vi "ViewData.vi"(7 "LabVIEW Web Service Request":refnum<class "Web Request.lvclass">) -> ()   [LabVIEW 2019]
uses:
  private/SendOutputDataState.ctl
  MobileAnalyzer/mainVIs/UIVIs/UIOutput.ctl
  MobileAnalyzer/mainVIs/analyzeAccelerationDataVIs/AccelerationDataFrames.ctl
  MobileAnalyzer/mainVIs/communicateWebServicesVIs/WebServicesData.ctl
  <vilib>/dex/Stream Element Allocation Mode.ctl
  <vilib>/wsapi/Web Request.lvclass
panel:
  # "Use the Web Service Request input terminal to call the VIs on the Web Services palette. Do not remove it from the connector pane unless you don't need access to the palette."
  # "Each additional control wired to the connector pane will be available as an input in the URL. To include an indicator in terminal-mode output (the default setting), it must also be wired to the connector pane."
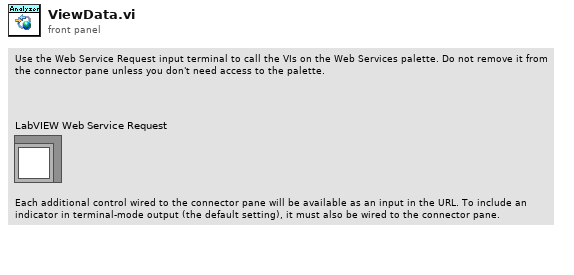
[diagram p1: front panel]
types:
  T1 = typedef "SendOutputDataState.ctl" = enum16{"Create analyzer endpoint", "Send output data", "End", "Init"}
  T2 = typedef "WebServicesData.ctl" = cluster{"AccelerationDataFrames":T3, "UIOutput":T4}
  T3 = typedef "AccelerationDataFrames.ctl" = cluster{"AccelerationData":waveform(dbl)[], "Amplitudes":cluster{"f0":dbl, "df":dbl, "real part":dbl[]}[], "Phases":cluster{"f0":dbl, "df":dbl, "imaginary part":dbl[]}[]}
  T4 = typedef "UIOutput.ctl" = cluster{"Aquiring data":bool, "AnalyzerError":errorcluster, "FIFO overflow":bool, "Analyzing data":bool}
  T5 = typedef "Stream Element Allocation Mode.ctl" = u32
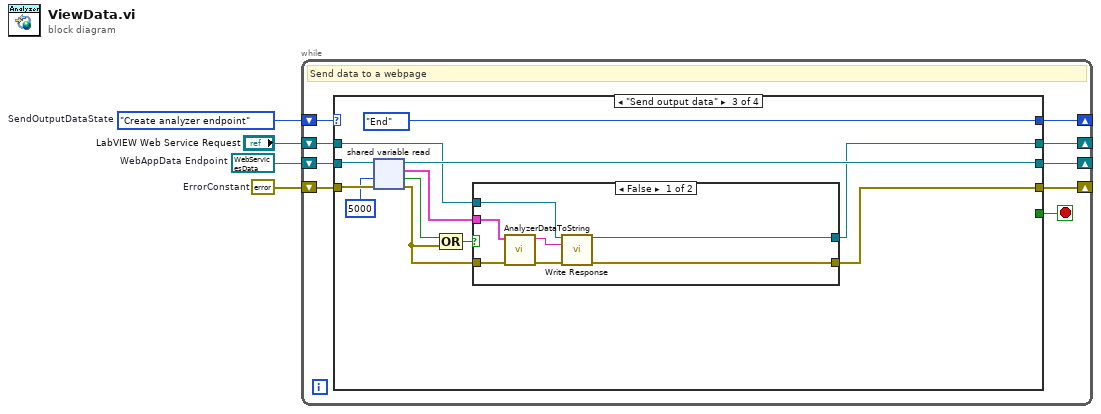
[diagram p0: block diagram]
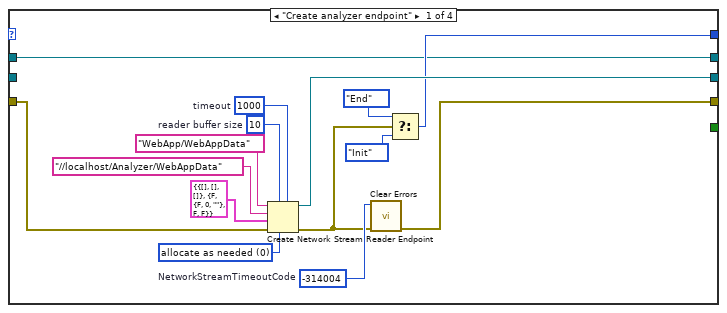
[diagram p2: hidden frame]
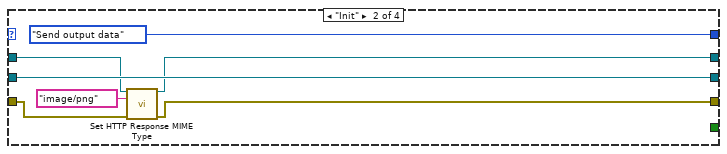
[diagram p3: hidden frame]
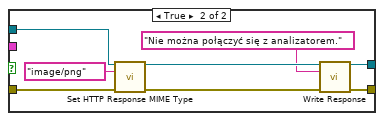
[diagram p4: hidden frame]
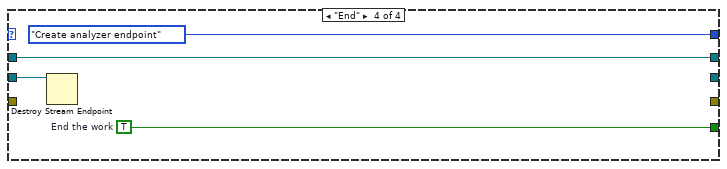
[diagram p5: hidden frame]
diagram:
  w2 = errorcluster {"status"=FALSE, "code"=0, "source"=""}  # ErrorConstant
  w3 = refnum<k21> refnum  # WebAppData Endpoint
  w4 = SendOutputDataState."Create analyzer endpoint"  # SendOutputDataState
  n1 = while {
    shift-right: [w12] -> _
    shift-left: w4 -> [w13]
    shift-right: [w9] -> _
    shift-left: w3 -> [w8]
    shift-right: [w10] -> _
    shift-left: w2 -> [w11]
    shift-right: [w5] -> _
    shift-left: "LabVIEW Web Service Request" -> [w6]
    stop <- w7 stop-if-true
    # "Send data to a webpage"
    n2 = case shown="\"Send output data\"" w13 {
      tunnel: [w16 SendOutputDataState."Send output data" ("f") SendOutputDataState."End" ("SendOutputDataState") SendOutputDataState."Create analyzer endpoint" ("f")] -> w12
      tunnel: w6 -> [w14 w32 w41 w63]
      tunnel: w11 -> [w25 w30 w46 _]
      tunnel: [w19 w31 w38 _] -> w10
      tunnel: [w24 w34 w44 _] -> w9
      tunnel: w8 -> [_ w34 w47 w66]
      tunnel: [_ _ _ w65] -> w7
      tunnel: [w14 w29 w36 w63] -> w5
      frame "Create analyzer endpoint" {
        w20 = -314004  # NetworkStreamTimeoutCode
        w21 = T5 0 items=["allocate as needed", "pre-allocate"] ("element allocation mode")
        w22 = 1000  # timeout
        w23 = 10  # reader buffer size
        n3 = Create Network Stream Reader Endpoint(5:w22, 6:w21, 7:w23, 8:w25, 9:T2 {"AccelerationDataFrames"={"AccelerationData"=[], "Amplitudes"=[], "Phases"=[]}, "UIOutput"={"Aquiring data"=FALSE, "AnalyzerError"={"status"=FALSE, "code"=0, "source"=""}, "FIFO overflow"=FALSE, "Analyzing data"=FALSE}} ("WebServicesData"), 10:"//localhost/Analyzer/WebAppData" ("writer name"), 11:"WebApp/WebAppData" ("reader name")) -> (0:w18:errorcluster, 3:w24:refnum<k21>)
        n4 = call <vilib>:"Clear Errors.vi"("error in (no error)"=w18, "specific error code to clear (0: all)"=w20) -> ("error out"=w19:errorcluster)  [unwired: 4 in, 1 out]
        n5 = Select(t=SendOutputDataState."End", s=w18, f=SendOutputDataState."Init") -> (s? t:f=w16:T1)
      }
      frame "Init" {
        n6 = call <vilib>:"Set HTTP Response MIME Type.vi"("LabVIEW Web Service Request"=w32, "MIME type (text/html)"="image/png", "error in (no error)"=w30) -> ("LabVIEW Web Service Request out"=w29:refnum<class "Web Request.lvclass">, "error out"=w31:errorcluster)  [unwired: 11 in]
      }
      frame "Send output data" {
        n7 = shared-variable-read(w47, w46, 5000 ("timeout ms (-1)")) -> (w44:refnum<k21>, w40:errorcluster, w39:bool, w43:T2)
        n8 = Compound Arithmetic op=OR(w39, w40) -> (w42:bool)
        n9 = case shown="False" w42 {
          tunnel: w43 -> [w50 _]
          tunnel: w41 -> [w51 w59]
          tunnel: w40 -> [w54 w60]
          tunnel: [w49 w62] -> w38
          tunnel: [w48 w55] -> w36
          frame False {
            n10 = call "AnalyzerDataToString.vi"("ErrorIn"=w54, "WebServicesData"=w50) -> ("ErrorOut"=w53:errorcluster, "String"=w52:string)  [unwired: 8 in]
            n11 = call <vilib>:"Write Response.vi"("LabVIEW Web Service Request"=w51, "response string"=w52, "error in (no error)"=w53) -> ("LabVIEW Web Service Request out"=w48:refnum<class "Web Request.lvclass">, "error out"=w49:errorcluster)  [unwired: 11 in]
          }
          frame True {
            n12 = call <vilib>:"Set HTTP Response MIME Type.vi"("LabVIEW Web Service Request"=w59, "MIME type (text/html)"="image/png", "error in (no error)"=w60) -> ("LabVIEW Web Service Request out"=w58:refnum<class "Web Request.lvclass">, "error out"=w56:errorcluster)  [unwired: 11 in]
            n13 = call <vilib>:"Write Response.vi"("LabVIEW Web Service Request"=w58, "response string"="Nie można połączyć się z analizatorem.", "error in (no error)"=w56) -> ("LabVIEW Web Service Request out"=w55:refnum<class "Web Request.lvclass">, "error out"=w62:errorcluster)  [unwired: 11 in]
          }
        }
      }
      frame "End" {
        w65 = TRUE  # End the work
        n14 = Destroy Stream Endpoint(11:w66) -> ()  [unwired: 1 in, 1 out]
      }
    }
  }
